vi "Add.vi"(8 "error in (no error)":errorcluster, 11 "Progress in":refnum<class "Progress.lvclass">) -> (0 "error out":errorcluster, 3 "Progress out":refnum<class "Progress.lvclass">)   [LabVIEW 2021, in "Progress.lvlib" / "Progress.lvclass"]
uses:
  Progress.lvclass
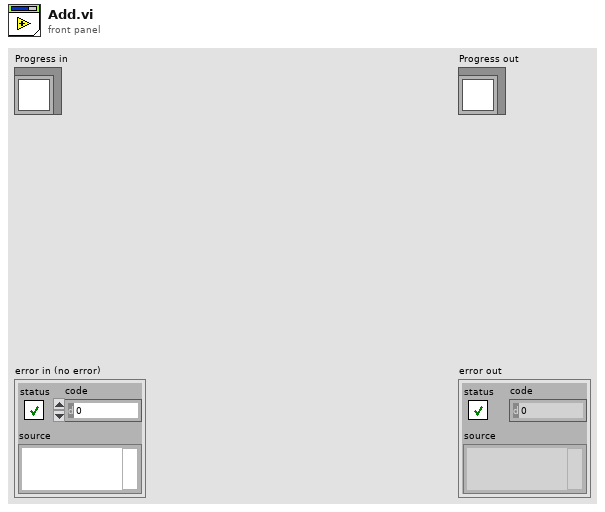
[diagram p1: front panel]
types:
  T1 = typedef "Progress.lvlib/Progress.lvclass/Data.ctl" = cluster{"SlideRefnum":refnum<vi>, "ProgressValue":u64, "NbElement":u64, "Caption":string, "UINotifier":refnum<notifier>, "StopUI":refnum<user-event>}
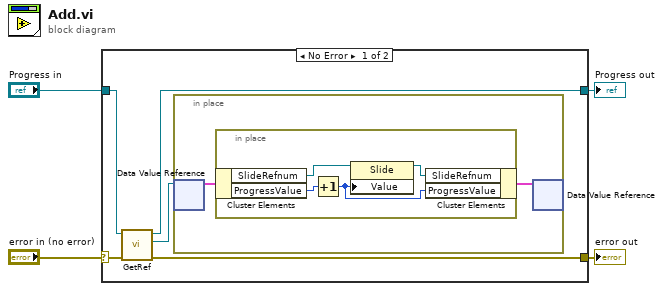
[diagram p0: block diagram]
diagram:
  n1 = case shown="No Error" "error in (no error)" {
    selector: "error in (no error)" -> [w8 w17]
    tunnel: [w7 w17] -> w3
    tunnel: [w5 w16] -> w1
    tunnel: "Progress in" -> [w9 w16]
    frame No Error {
      n2 = call "GetRef.vi"("error in (no error)"=w8, "Progress in"=w9) -> ("error out"=w7:errorcluster, "ref"=w6:refnum<data-value>, "Progress out"=w5:refnum<class "Progress.lvclass">)  [unwired: 7 in]
      n3 = in-place {
        n4 = in-place-dvr #1(w6) -> (w11:T1)  [unwired: 1 out]
        n5 = in-place {
          n6 = in-place-cluster #2(w11) -> ("SlideRefnum"=w15:refnum<vi>, "ProgressValue"=w13:u64)
          n7 = Increment(x=w13) -> (x+1=w12:u64)
          n8 = property class="Slide"(reference=w15, "Value"=w12) -> (reference out=w14:refnum<vi>)  [unwired: 1 in, 1 out]
          n9 = in-place-cluster #2("SlideRefnum"=w14, "ProgressValue"=w12) -> (w10:T1)
        }
        n10 = in-place-dvr #1(w10) -> ()  [unwired: 2 out]
      }
    }
    frame Error {
    }
  }
  "error out" <- w3
  "Progress out" <- w1
